vi "Pilot Analyze.vi"(5 "JoystickDevRef":T1) -> (3 "x":dbl, 4 "y":dbl, 6 "close arms":bool, 8 "second preperation":bool, 10 "pull wire":bool, 13 "open arms":bool, 14 "Shut Down System":bool, 15 "Slow Drive":bool)   [LabVIEW 2012]
uses:
  <vilib>/Rock Robotics/WPI/Joystick/WPI_JoystickDevRef.ctl
  <vilib>/Rock Robotics/WPI/Joystick/WPI_JoystickDeviceEnum.ctl
  BotStatus.vi
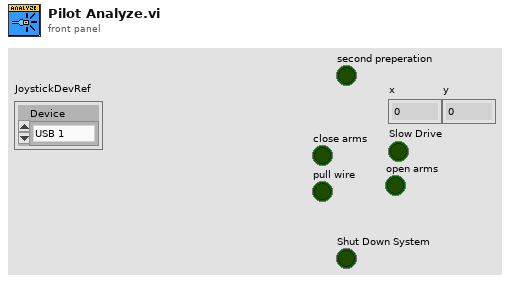
[diagram p1: front panel]
types:
  T1 = typedef "WPI_JoystickDevRef.ctl" = cluster{"Device":T2}
  T2 = typedef "WPI_JoystickDeviceEnum.ctl" = enum16{"USB 1", "USB 2", "USB 3", "USB 4", "Kinect 1", "Kinect 2"}
  T3 = typedef "WPI_JoystickButtonState.ctl" = cluster{"Button 1":bool, "Button 2":bool, "Button 3":bool, "Button 4":bool, "Button 5":bool, "Button 6":bool, "Button 7":bool, "Button 8":bool, "Button 9":bool, "Button 10":bool, "Button 11":bool, "Button 12":bool}
  T4 = cluster{"axis 1 (x)":dbl, "axis 2 (y)":dbl, "axis 3 (throttle)":dbl, "axis 4":dbl, "axis 5":dbl, "axis 6":dbl}
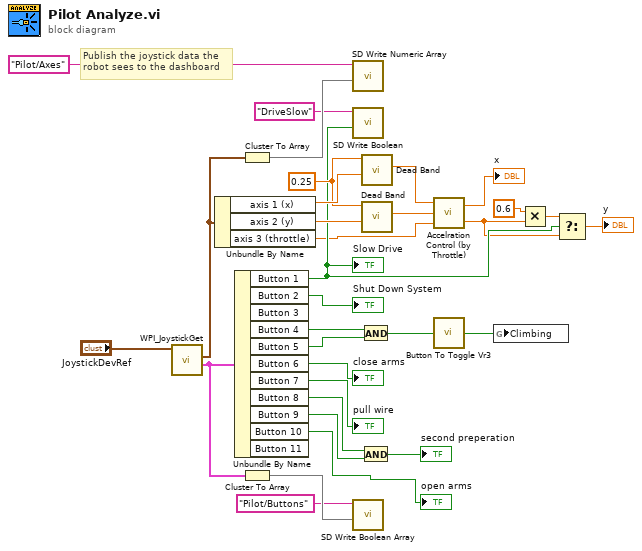
[diagram p0: block diagram]
diagram:
  w25 = 0.25 ("Dead Band")
  # "Publish the joystick data the\nrobot sees to the dashboard"
  n1 = call <vilib>:"WPI_JoystickGet.vi"("JoystickDevRef"="JoystickDevRef") -> ("Buttons"=w17:T3, "Axes"=w18:T4)  [unwired: 4 in, 1 out]
  n2 = Unbundle By Name(w18) -> ("axis 1 (x)"=w29:dbl, "axis 2 (y)"=w27:dbl, "axis 3 (throttle)"=w14:dbl)
  n3 = Unbundle By Name(w17) -> ("Button 1"=w16:bool, "Button 2"=→"Shut Down System":bool, "Button 4"=w8:bool, "Button 5"=w7:bool, "Button 6"=→"close arms":bool, "Button 7"=→"pull wire":bool, "Button 8"=w4:bool, "Button 9"=w3:bool, "Button 10"=→"open arms":bool)  [unwired: 2 out]
  "Slow Drive" <- w16
  n4 = Cluster To Array(cluster=w18) -> (array=w20:dbl[])
  n5 = Cluster To Array(cluster=w17) -> (array=w22:bool[])
  n6 = call <vilib>:"SD Write Numeric Array.vi"("Numeric Array"=w20, "Name"="Pilot/Axes") -> ()  [unwired: 8 in, 2 out]
  n7 = call <vilib>:"SD Write Boolean.vi"("Boolean"=w16, "Name"="DriveSlow") -> ()  [unwired: 8 in, 2 out]
  n8 = call <vilib>:"SD Write Boolean Array.vi"("Boolean Array"=w22, "Name"="Pilot/Buttons") -> ()  [unwired: 8 in, 2 out]
  n9 = And(x=w8, y=w7) -> (x .and. y?=w6:bool)
  n10 = And(x=w4, y=w3) -> (x .and. y?=→"second preperation":bool)
  n11 = call "Dead Band.vi"("Axis In"=w29, "Dead Band"=w25) -> ("Axis Out"=w28:dbl)  [unwired: 9 in]
  n12 = call "Dead Band.vi"("Axis In"=w27, "Dead Band"=w25) -> ("Axis Out"=w26:dbl)  [unwired: 9 in]
  n13 = call "Accelration Control (by Throttle).vi"("acc"=w14, "Yinput"=w26, "Xinput"=w28) -> ("Youtput"=w12:dbl, "Xoutput"=→"x":dbl)
  n14 = call "Button To Toggle Vr3.vi"("InValue"=w6) -> ("Result"=w5:bool)
  n15 = global write "BotStatus.vi" "Climbing"(w5) -> ()
  n16 = Multiply(x=0.6 ("y"), y=w12) -> (x*y=w24:dbl)
  n17 = Select(t=w24, s=w16, f=w12) -> (s? t:f=→"y":dbl)
